vi "Operate.vi"(8 "error in (no error)":errorcluster, 11 "Subtract in":refnum<class "Subtract.lvclass">) -> (0 "error out":errorcluster, 3 "Subtract out":refnum<class "Subtract.lvclass">)   [LabVIEW 2020, in "Subtract.lvclass"]
doc: "This method is used in child class which is used to perform subtraction operation"
uses:
  Subtract.lvclass
  D:/labview/Assignment 24/Math Operations/Math Operations.lvclass
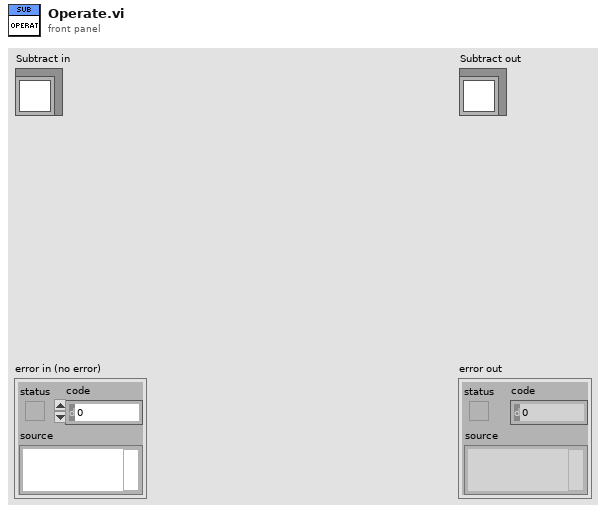
[diagram p1: front panel]
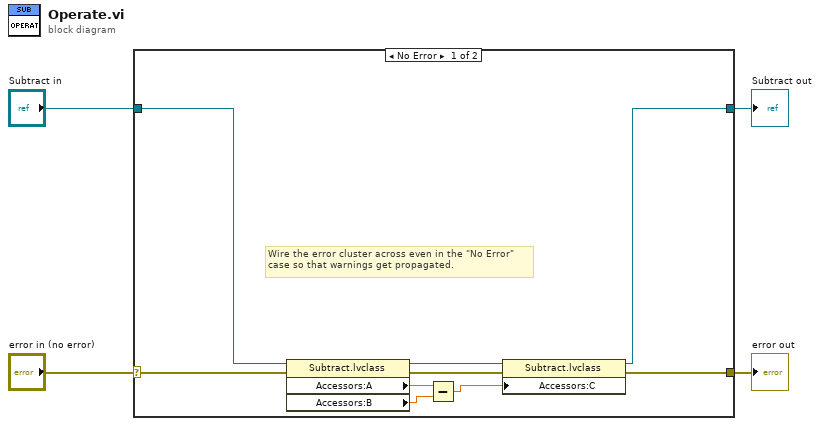
[diagram p0: block diagram]
diagram:
  n1 = case shown="No Error" "error in (no error)" {
    selector: "error in (no error)" -> [w12 w15]
    tunnel: [w8 w15] -> w3
    tunnel: [w5 w14] -> w1
    tunnel: "Subtract in" -> [w13 w14]
    frame No Error {
      # "Wire the error cluster across even in the \"No Error\"\ncase so that warnings get propagated."
      n2 = property class="Subtract.lvclass"(reference=w13, error in=w12) -> (reference out=w7:refnum<class "Subtract.lvclass">, error out=w9:errorcluster, "Accessors:A"=w11:dbl, "Accessors:B"=w10:dbl)
      n3 = Subtract(x=w11, y=w10) -> (x-y=w6:dbl)
      n4 = property class="Subtract.lvclass"(reference=w7, error in=w9, "Accessors:C"=w6) -> (reference out=w5:refnum<class "Subtract.lvclass">, error out=w8:errorcluster)
    }
    frame Error {
    }
  }
  "error out" <- w3
  "Subtract out" <- w1
